vi "Test controller module.vi"(8 "error in (no error)":errorcluster) -> (0 "error out":errorcluster)   [LabVIEW 2016]
uses:
  Controls/Test controller modes.ctl
  Controls/Queue modes.ctl
  Controls/State control cluster.ctl
  Controls/States.ctl
  Actuator/Controls/Actuator fgv modes.ctl
  Actuator/Controls/Command cluster.ctl
  Actuator/Controls/Command list.ctl
  Controls/staus modes.ctl
  Webcam/Controls/Camera queue.ctl
  Webcam/Controls/Camera states.ctl
  DAQ/Controls/DAQ queue.ctl
  DAQ/Controls/Queue states.ctl
  Controls/data modes.ctl
  <vilib>/Utility/config.llb/NI_LVConfig.lvlib
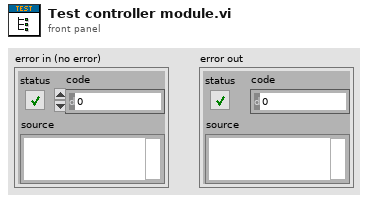
[diagram p1: front panel]
types:
  T1 = typedef "Queue modes.ctl" = enum16{"Initialise", "Destroy", "Get"}
  T2 = typedef "Test controller modes.ctl" = enum16{"Idle", "Test setup", "Check connections", "Populate FGV", "Load actuator settings", "Snap image", "Start move", "Start LC capture", "Wait", "Monitor", "Stop LC capture", "Save LC data", "Save Ivium data", "Save data"}
  T3 = typedef "References.ctl" = cluster{"Tab Control":refnum<vi>, "Logo 1":refnum<vi>, "Logo 2":refnum<vi>, "Connect Actuator":refnum<vi>, "LIVE DATA":refnum<vi>, "Speed":refnum<vi>, "Home position":refnum<vi>, "Limit position":refnum<vi>, "Trigger":refnum<vi>, "Current position":refnum<vi>, "Connect Camera":refnum<vi>, "TEST DATA":refnum<vi>, "LIVE DATA Force":refnum<vi>, "Connect DAQ":refnum<vi>, "Initialised":refnum<vi>, "Test":refnum<vi>}
  T4 = typedef "UEs.ctl" = cluster{"Read position":refnum<user-event>, "Check home":refnum<user-event>, "Record":refnum<user-event>, "Abort controller":refnum<user-event>, "Remote test":refnum<user-event>, "Test setup":refnum<user-event>, "Conditional wait":refnum<user-event>, "Abort move":refnum<user-event>, "Wait done":refnum<user-event>, "Send trigger":refnum<user-event>, "Initalising":refnum<user-event>, "Initalisation complete":refnum<user-event>}
  T5 = typedef "Command cluster.ctl" = cluster{"Command":T6, "data":variant}
  T6 = typedef "Command list.ctl" = enum16{"", "£nabort", "getaxisno", "£getserialno", "£nidentify", "&&£setnlimit", "&£nm", "&£snv", "&£speed", "£np", "£ncal"}
  T7 = typedef "Actuator fgv modes.ctl" = enum16{"Initalise", "COM", "Limit", "Speed", "Home", "Get"}
  T8 = typedef "State control cluster.ctl" = cluster{"State":T9, "Data":variant}
  T9 = typedef "States.ctl" = enum16{"Initialise", "Actuator connection", "Get info", "Send command", "Load method", "Run method", "Save test", "Setup", "Shutdown"}
  T10 = typedef "staus modes.ctl" = enum16{"Status", "Testing", "Webcam", "DAQ", "Actuator", "Initialise"}
  T11 = typedef "Camera queue.ctl" = cluster{"State":T12, "Data":variant}
  T12 = typedef "Camera states.ctl" = enum16{"Initialise", "Setup", "Connect", "Snap", "Close", "Shutdown"}
  T13 = typedef "DAQ queue.ctl" = cluster{"Sate":T14, "Data":variant}
  T14 = typedef "Queue states.ctl" = enum16{"Shutdown", "Save data", "Record", "Read", "Setup", "Zero", "Connect", "Initialise"}
  T15 = typedef "data modes.ctl" = enum16{"Initalise", "Status", "Process", "Add load", "Add position"}
  T16 = enum16{"open", "replace", "create", "open or create", "replace or create", "replace or create with confirmation"}
  T17 = typedef "Test settings.ctl" = cluster{"Speed (mm/s)":dbl, "Position limit":bool, "Position limit (mm)":dbl, "Load limit":bool, "Load limit (N)":dbl, "No. of repeats":u16, "Test identifier":string, "Time wait":bool, "Wait time (s)":dbl, "Trigger wait":bool, "Send trigger":bool, "Test notes":string, "Snap intervals":bool, "Time interval (s)":dbl}
  T18 = typedef "NI_LVConfig.lvlib/Config Data RefNum.ctl" = refnum<k1>
  T19 = typedef "Default settings.ctl" = cluster{"COM port":refnum<visa-resource-name>, "Home pos":dbl, "Speed":dbl, "Limit stop":dbl}
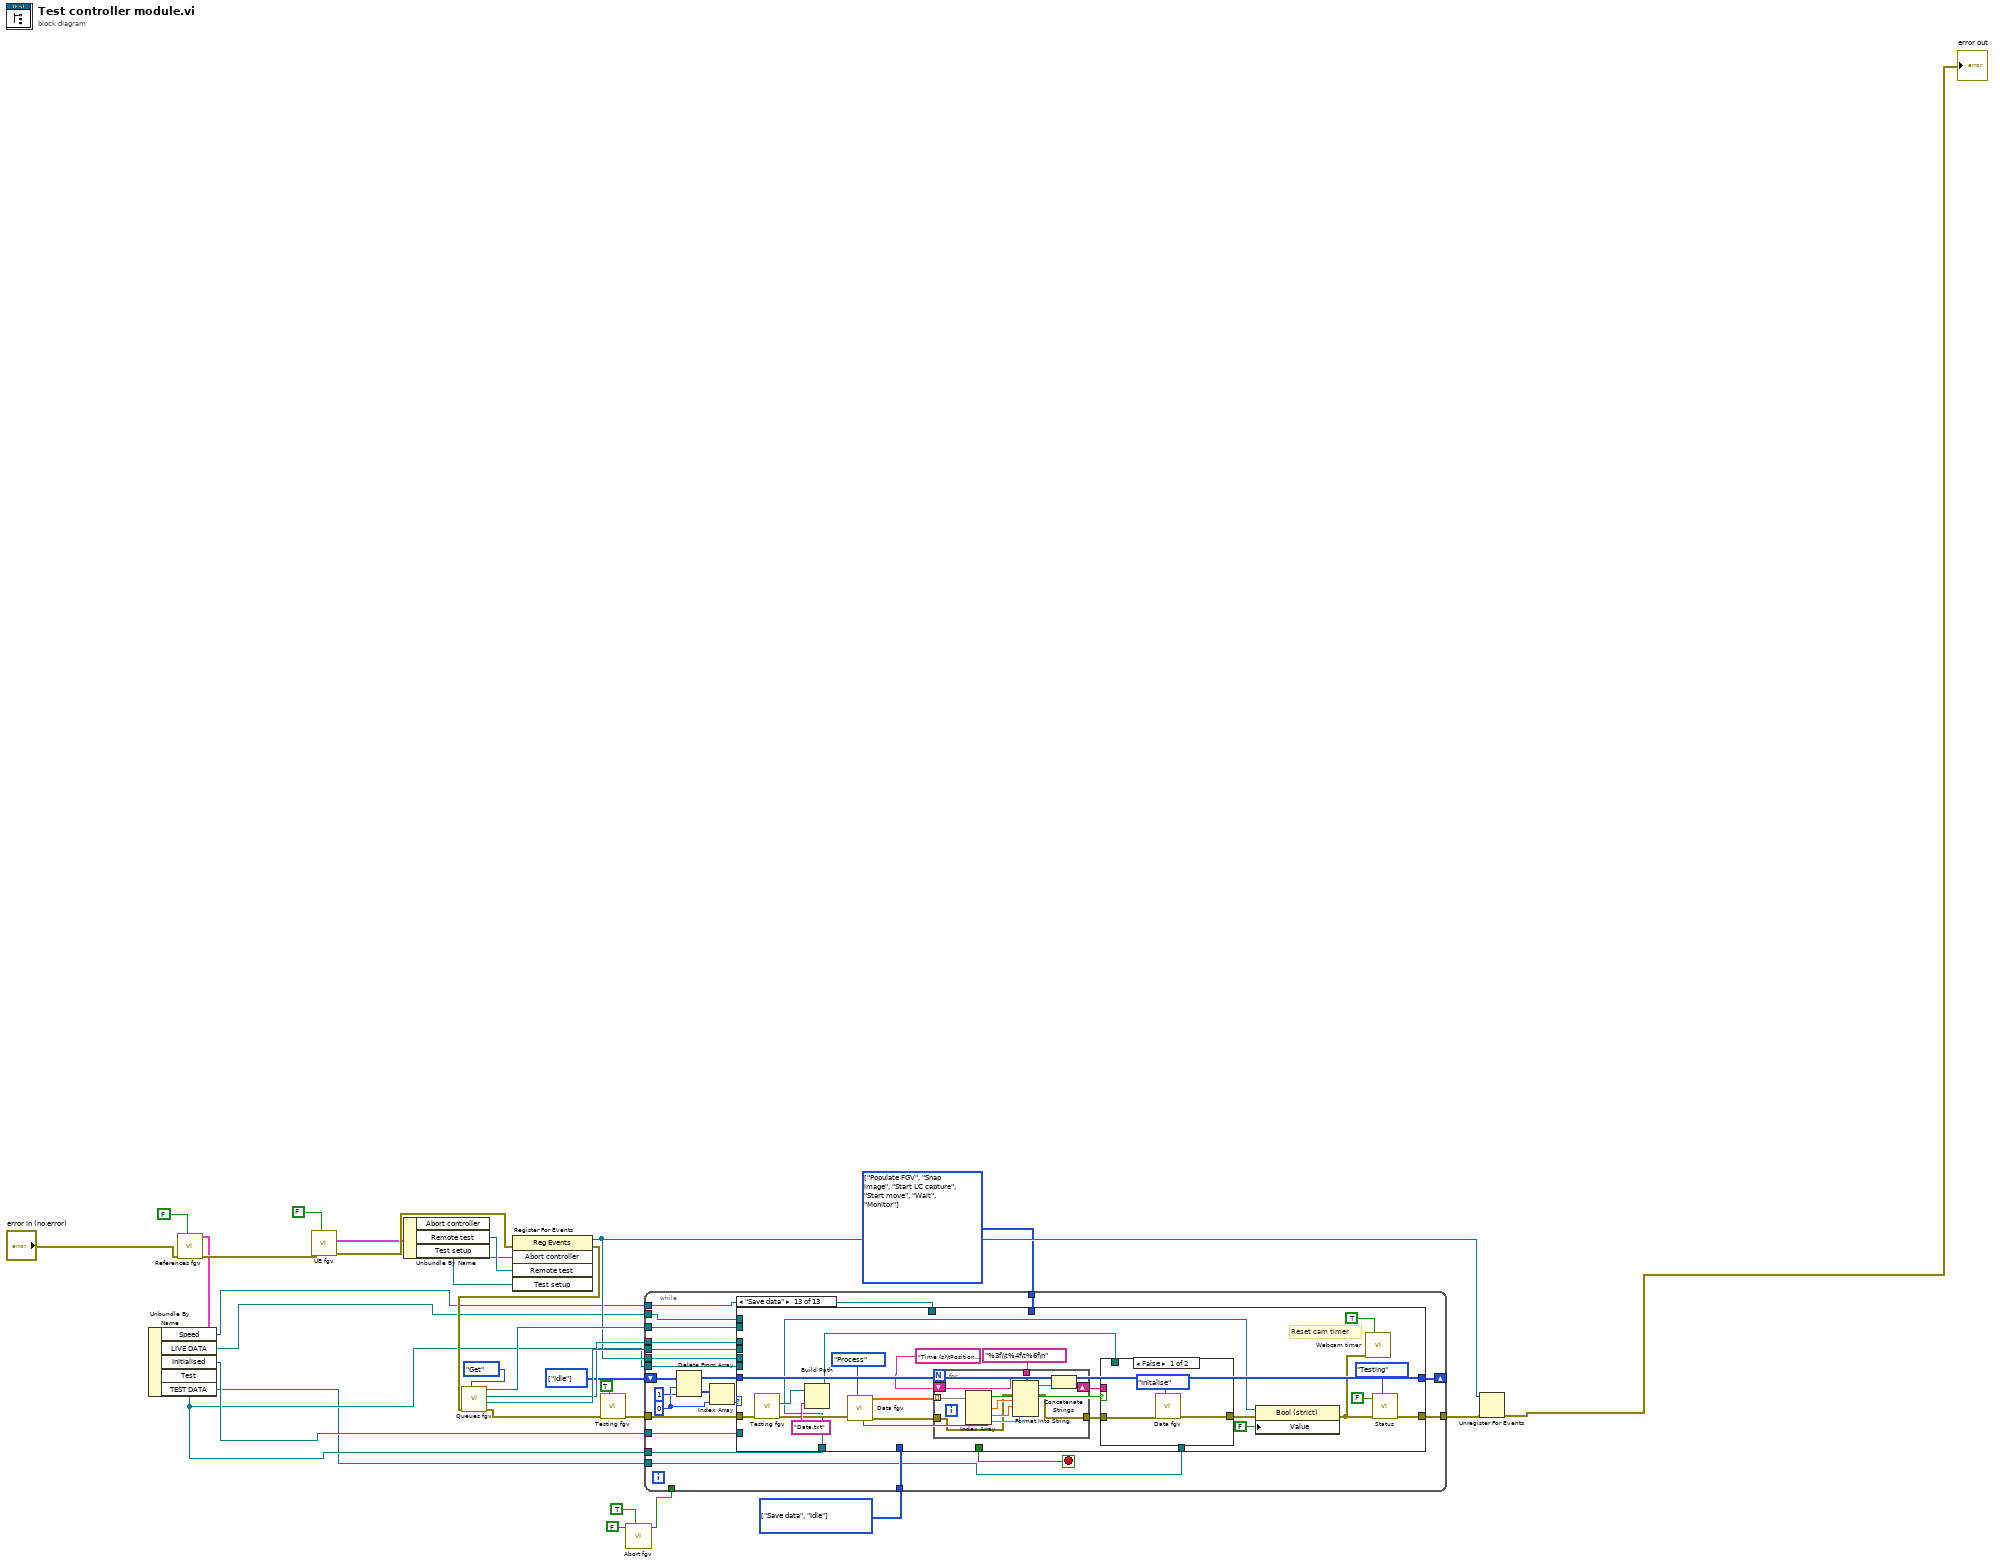
[diagram p0: block diagram]
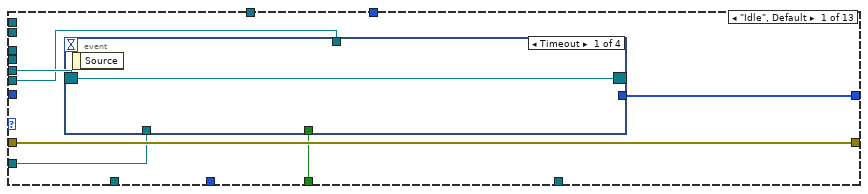
[diagram p2: hidden frame]
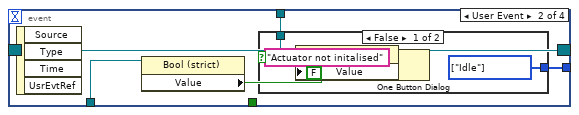
[diagram p3: hidden frame]
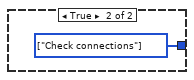
[diagram p4: hidden frame]
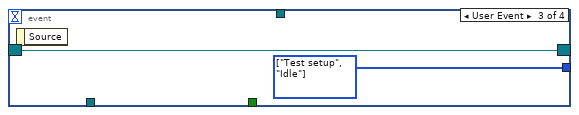
[diagram p5: hidden frame]
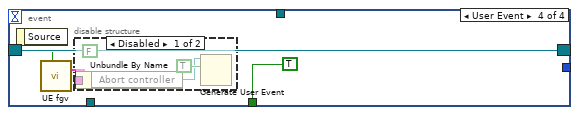
[diagram p6: hidden frame]
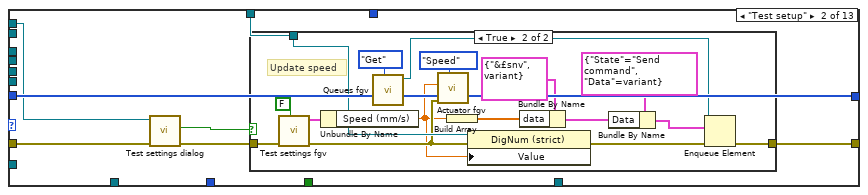
[diagram p8: hidden frame]
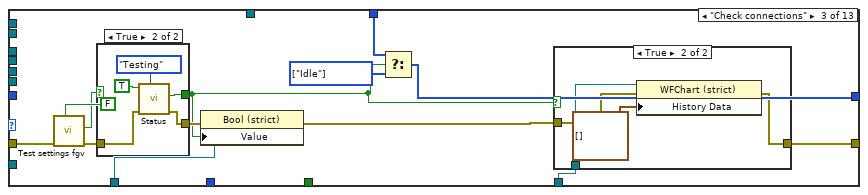
[diagram p10: hidden frame]
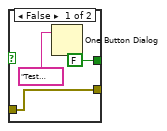
[diagram p12: hidden frame]
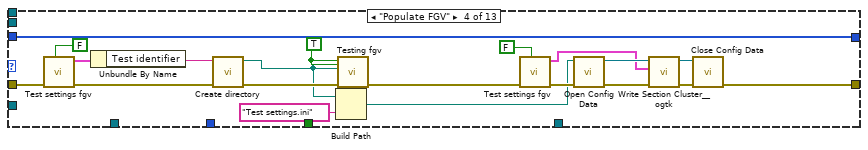
[diagram p13: hidden frame]
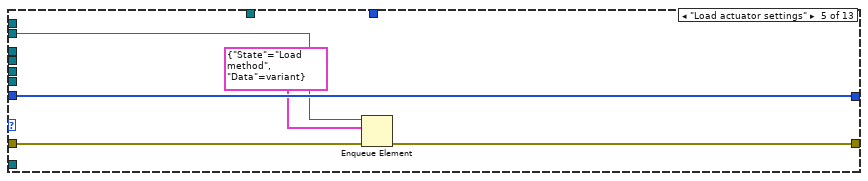
[diagram p14: hidden frame]
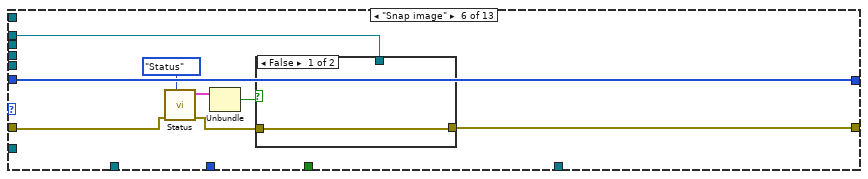
[diagram p15: hidden frame]
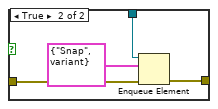
[diagram p16: hidden frame]
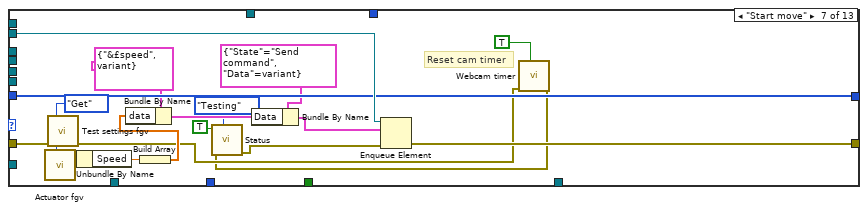
[diagram p17: hidden frame]
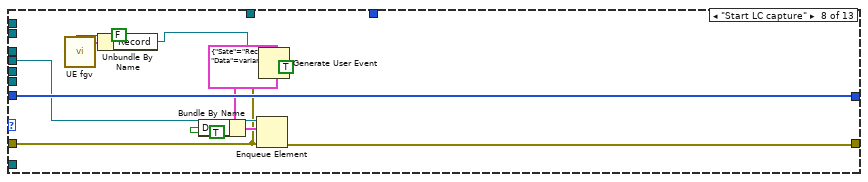
[diagram p18: hidden frame]
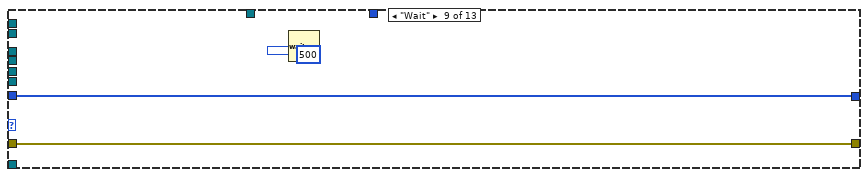
[diagram p19: hidden frame]
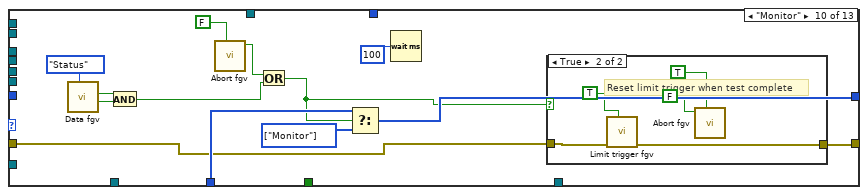
[diagram p20: hidden frame]
diagram:
  w15 = T2[] [enum."Save data", enum."Idle"] items=["Idle", "Test setup", "Check connections", "Populate FGV", "Load actuator settings", "Snap image", "Start move", "Start LC capture", "Wait", "Monitor", "Stop LC capture", "Save LC data", "Save Ivium data", "Save data"]
  w13 = T2[] [enum."Idle"] items=["Idle", "Test setup", "Check connections", "Populate FGV", "Load actuator settings", "Snap image", "Start move", "Start LC capture", "Wait", "Monitor", "Stop LC capture", "Save LC data", "Save Ivium data", "Save data"]
  w14 = T2[] [enum."Populate FGV", enum."Snap image", enum."Start LC capture", enum."Start move", enum."Wait", enum."Monitor"] items=["Idle", "Test setup", "Check connections", "Populate FGV", "Load actuator settings", "Snap image", "Start move", "Start LC capture", "Wait", "Monitor", "Stop LC capture", "Save LC data", "Save Ivium data", "Save data"]
  n1 = call "References fgv.vi"("Set?"=FALSE, "error in (no error)"="error in (no error)") -> ("error out"=w12:errorcluster, "Cluster"=w9:T3)  [unwired: 8 in]
  n2 = Unbundle By Name(w9) -> ("Speed"=w8:refnum<vi>, "LIVE DATA"=w7:refnum<vi>, "Initialised"=w6:refnum<vi>, "Test"=w5:refnum<vi>, "TEST DATA"=w4:refnum<vi>)
  n3 = call "UE fgv.vi"("Set?"=FALSE, "error in (no error)"=w12) -> ("error out"=w31:errorcluster, "UEs"=w27:T4)  [unwired: 7 in, 1 out]
  n4 = Unbundle By Name(w27) -> ("Abort controller"=w28:refnum<user-event>, "Remote test"=w29:refnum<user-event>, "Test setup"=w30:refnum<user-event>)
  n5 = register-events(error in=w31, w28, w29, w30) -> (reference out=w20:refnum<event-registration>, error out=w32:errorcluster)  [unwired: 1 in]
  n6 = call "Queues fgv.vi"("Modes"=Queue_modes."Get", "error in (no error)"=w32) -> ("error in (no error) 2"=w25:errorcluster, "DAQ"=w24:refnum<queue>, "Camera"=w23:refnum<queue>, "Ivium"=w22:refnum<queue>)  [unwired: 6 in]
  n7 = call "Testing fgv.vi"("Populate"=TRUE, "error in (no error)"=w25) -> ("error out"=w17:errorcluster)  [unwired: 7 in, 2 out]
  n8 = call "Abort fgv.vi"("Set?"=TRUE, "Value"=FALSE) -> ("Value 2"=w1:bool)  [unwired: 9 in]
  n9 = while {
    shift-right: [w49] -> _
    shift-left: w13 -> [w54]
    tunnel: w14 -> [w48]
    tunnel: w22 -> [w47]
    tunnel: w23 -> [w44]
    tunnel: [w46] -> w18
    tunnel: w17 -> [w45]
    tunnel: w15 -> [w43]
    tunnel: w24 -> [w41]
    tunnel: w20 -> [w40]
    tunnel: w5 -> [w38]
    tunnel: w7 -> [w37]
    tunnel: w8 -> [w36]
    tunnel: w6 -> [w35]
    tunnel: w5 -> [w34]
    tunnel: w4 -> [w33]
    tunnel: w1 -> [_]
    stop <- w39 stop-if-true
    w42 = 0 ("index")
    n10 = Delete From Array(array=w54, length=1, index=w42) -> (deleted portion=w52:T2[], array with subset deleted=w50:T2[])
    n11 = Index Array(array=w52, index=w42) -> (element=w51:T2)
    n12 = case shown="\"Save data\"" w51 {
      tunnel: w50 -> [_ w87 _ w150 w155 w162 w184 w197 w199 _ w230 w241 w263]
      tunnel: [w60 w87 w116 w150 w155 w162 w184 w197 w199 w210 w230 w241 w263] -> w49
      tunnel: w48 -> [_ _ w117 _ _ _ _ _ _ _ _ _ _]
      tunnel: w47 -> [_ _ _ _ w154 _ w185 _ _ _ _ _ _]
      tunnel: [w59 w82 w107 w131 w153 w163 w186 w192 w198 w205 w229 w239 w247] -> w46
      tunnel: w45 -> [w59 w86 w112 w147 w152 w158 w182 w191 w198 w206 w224 w236 w262]
      tunnel: w44 -> [_ _ _ _ _ w161 _ _ _ _ _ _ _]
      tunnel: w43 -> [_ _ _ _ _ _ _ _ _ w211 _ _ _]
      tunnel: w41 -> [_ _ _ _ _ _ _ w196 _ _ w228 w240 _]
      tunnel: w40 -> [w58 _ _ _ _ _ _ _ _ _ _ _ _]
      tunnel: [w57 _ _ _ _ _ _ _ _ _ _ _ _] -> w39
      tunnel: w38 -> [_ _ w114 _ _ _ _ _ _ _ _ _ w249]
      tunnel: w37 -> [_ w85 _ _ _ _ _ _ _ _ _ _ _]
      tunnel: w36 -> [_ w81 _ _ _ _ _ _ _ _ _ _ _]
      tunnel: w35 -> [w56 _ _ _ _ _ _ _ _ _ _ _ _]
      tunnel: w34 -> [w55 _ _ _ _ _ _ _ _ _ _ _ _]
      tunnel: w33 -> [_ _ w105 _ _ _ _ _ _ _ _ _ _]
      frame "Idle", Default {
        n13 = event shown="[0] Timeout" {
          selector: w58 -> [w61 w65 w73 w76]
          dyn-events: [w61 w65 w73 w76] -> _
          timeout: _ -> [_ _ _ _]
          tunnel: [_ w66 w72 _] -> w60
          tunnel: [_ _ _ TRUE] -> w57
          tunnel: w56 -> [_ w64 _ _]
          tunnel: w55 -> [_ w62 _ _]
          event Timeout {
            n14 = event-data() -> ()  [unwired: 1 in, 1 out]
          }
          event User Event {
            n15 = event-data() -> ()  [unwired: 1 in, 4 out]
            n16 = property class="Bool (strict)"(reference=w64) -> ("Value"=w63:bool)  [unwired: 1 in, 2 out]
            n17 = case shown="False" w63 {
              tunnel: [w70 w71] -> w66
              tunnel: w62 -> [w67 _]
              frame False {
                w70 = T2[] [enum."Idle"] items=["Idle", "Test setup", "Check connections", "Populate FGV", "Load actuator settings", "Snap image", "Start move", "Start LC capture", "Wait", "Monitor", "Stop LC capture", "Save LC data", "Save Ivium data", "Save data"]
                n18 = property on="Property Node" class="Bool (strict)"(reference=w67, "Value"=FALSE ("Test")) -> ()  [unwired: 1 in, 2 out]
                n19 = One Button Dialog(message="Actuator not initalised") -> ()  [unwired: 1 in, 1 out]
              }
              frame True {
                w71 = T2[] [enum."Check connections"] items=["Idle", "Test setup", "Check connections", "Populate FGV", "Load actuator settings", "Snap image", "Start move", "Start LC capture", "Wait", "Monitor", "Stop LC capture", "Save LC data", "Save Ivium data", "Save data"]
              }
            }
          }
          event User Event {
            w72 = T2[] [enum."Test setup", enum."Idle"] items=["Idle", "Test setup", "Check connections", "Populate FGV", "Load actuator settings", "Snap image", "Start move", "Start LC capture", "Wait", "Monitor", "Stop LC capture", "Save LC data", "Save Ivium data", "Save data"]
            n20 = event-data() -> ()  [unwired: 1 in, 1 out]
          }
          event User Event {
            n21 = event-data() -> ()  [unwired: 1 in, 1 out]
            n22 = call "UE fgv.vi"("Set?"=FALSE) -> ("UEs"=w74:T4)  [unwired: 8 in, 2 out]
            n23 = disable-structure shown="Disabled" {
              disable-tunnel: w74 -> [w79 _]
              frame Disabled {
                n24 = Unbundle By Name(w79) -> ("Abort controller"=w78:refnum<user-event>)
                n25 = Generate User Event(user event=w78, event data cluster=TRUE ("event data")) -> ()  [unwired: 2 in, 2 out]
              }
              frame Enabled {
              }
            }
          }
        }
      }
      frame "Test setup" {
        n26 = call "Test settings dialog.vi"("error in (no error)"=w86, "LIVE DATA 3"=w85) -> ("error out"=w83:errorcluster, "Confirmed"=w84:bool)  [unwired: 7 in, 1 out]
        n27 = case shown="True" w84 {
          tunnel: w83 -> [w88 w101]
          tunnel: [w88 w96] -> w82
          tunnel: w81 -> [_ w95]
          frame False {
          }
          frame True {
            # "Update speed"
            n28 = call "Test settings fgv.vi"("Set?"=FALSE, "error in (no error)"=w101) -> ("error out"=w94:errorcluster, "Test settings out"=w99:T17)  [unwired: 7 in, 1 out]
            n29 = Unbundle By Name(w99) -> ("Speed (mm/s)"=w90:dbl)
            n30 = call "Queues fgv.vi"("Modes"=Queue_modes."Get") -> ("Ivium"=w91:refnum<queue>)  [unwired: 7 in, 3 out]
            n31 = call "Actuator fgv.vi"("Enum"=Actuator_fgv_modes."Speed", "error in (no error)"=w94, "Data"=w90) -> ()  [unwired: 7 in, 2 out]
            n32 = Build Array(w90) -> (w89:dbl[])
            n33 = property class="DigNum (strict)"(reference=w95, error in=w94, "Value"=w90) -> (error out=w93:errorcluster)  [unwired: 1 out]
            n34 = Bundle By Name(cluster=T5 {"Command"=enum."&£snv", "data"=variant} ("Cluster"), "data"=w89) -> (w97:T5)
            n35 = Bundle By Name(cluster=T8 {"State"=enum."Send command", "Data"=variant} ("element"), "Data"=w97) -> (w103:T8)
            n36 = Enqueue Element(queue=w91, element=w103, error in (no error)=w93) -> (error out=w96:errorcluster)  [unwired: 1 in, 2 out]
          }
        }
      }
      frame "Check connections" {
        w115 = T2[] [enum."Idle"] items=["Idle", "Test setup", "Check connections", "Populate FGV", "Load actuator settings", "Snap image", "Start move", "Start LC capture", "Wait", "Monitor", "Stop LC capture", "Save LC data", "Save Ivium data", "Save data"] ("f")
        n37 = call "Test settings fgv.vi"("Set?"=FALSE, "error in (no error)"=w112) -> ("error out"=w111:errorcluster, "Settings selected?  out"=w109:bool)  [unwired: 7 in, 1 out]
        n38 = case shown="True" w109 {
          tunnel: [FALSE ("Testing") w130] -> w106
          tunnel: [w124 w129] -> w113
          tunnel: w111 -> [w124 w128]
          frame False {
            n39 = One Button Dialog(message="Test settings not selected.") -> ()  [unwired: 1 in, 1 out]
          }
          frame True {
            n40 = call "Status.vi"("Mode"=staus_modes."Testing", "error in (no error)"=w128, "Data"=TRUE) -> ("error out"=w129:errorcluster, "Testing"=w130:bool)  [unwired: 6 in, 1 out]
          }
        }
        n41 = property class="Bool (strict)"(reference=w114, error in=w113, "Value"=w106) -> (error out=w108:errorcluster)  [unwired: 1 out]
        n42 = Select(t=w117, s=w106, f=w115) -> (s? t:f=w116:T2[])
        n43 = case shown="True" w106 {
          tunnel: w108 -> [w118 w121]
          tunnel: [w118 w120] -> w107
          tunnel: w105 -> [_ w119]
          frame False {
          }
          frame True {
            n44 = property class="WFChart (strict)"(reference=w119, error in=w121, "History Data"=cluster{"Value":dbl, "data":dbl}[] []) -> (error out=w120:errorcluster)  [unwired: 1 out]
          }
        }
      }
      frame "Populate FGV" {
        w148 = TRUE ("Populate")
        n45 = call "Test settings fgv.vi"("Set?"=FALSE, "error in (no error)"=w147) -> ("error out"=w146:errorcluster, "Test settings out"=w144:T17)  [unwired: 7 in, 1 out]
        n46 = Unbundle By Name(w144) -> ("Test identifier"=w143:string)
        n47 = call "Create directory.vi"("error in (no error)"=w146, "Identifier 1"=w143) -> ("error out"=w149:errorcluster, "created path"=w135:path)  [unwired: 8 in]
        n48 = Build Path(base path=w135, name or relative path="Test settings.ini") -> (appended path=w133:path)
        n49 = call "Testing fgv.vi"("Populate"=w148, "error in (no error)"=w149, "test dir In"=w135, "Testing? In"=w148) -> ("error out"=w132:errorcluster)  [unwired: 5 in, 2 out]
        n50 = call "Test settings fgv.vi"("Set?"=FALSE, "error in (no error)"=w132) -> ("error out"=w138:errorcluster, "Test settings out"=w139:T17)  [unwired: 7 in, 1 out]
        n51 = call <vilib>:"Open Config Data.vi"("error in (no error)"=w138, "configuration file path"=w133) -> ("error out"=w137:errorcluster, "refnum"=w141:T18)  [unwired: 7 in, 1 out]
        n52 = call "Write Section Cluster__ogtk.vi"("error in (no error)"=w137, "Section Formatted Cluster"=w139, "refnum"=w141) -> ("error out"=w136:errorcluster, "dup refnum"=w142:T18)  [unwired: 7 in]
        n53 = call <vilib>:"Close Config Data.vi"("error in (no error)"=w136, "refnum"=w142) -> ("error out"=w131:errorcluster)  [unwired: 8 in, 1 out]
      }
      frame "Load actuator settings" {
        n54 = Enqueue Element(queue=w154, element=T8 {"State"=enum."Load method", "Data"=variant} ("State control"), error in (no error)=w152) -> (error out=w153:errorcluster)  [unwired: 1 in, 2 out]
      }
      frame "Snap image" {
        n55 = call "Status.vi"("Mode"=staus_modes."Status", "error in (no error)"=w158) -> ("error out"=w157:errorcluster, "Connections"=w160:cluster{"Data":bool, "Data":bool, "Data":bool})  [unwired: 7 in, 1 out]
        n56 = Unbundle(w160) -> ("Data"=w159:bool)  [unwired: 2 out]
        n57 = case shown="False" w159 {
          tunnel: [w164 w168] -> w163
          tunnel: w157 -> [w164 w167]
          tunnel: w161 -> [_ w165]
          frame False {
          }
          frame True {
            n58 = Enqueue Element(queue=w165, element=T11 {"State"=enum."Snap", "Data"=variant}, error in (no error)=w167) -> (error out=w168:errorcluster)  [unwired: 1 in, 2 out]
          }
        }
      }
      frame "Start move" {
        # "Reset cam timer"
        n59 = call "Actuator fgv.vi"("Enum"=Actuator_fgv_modes."Get") -> ("Cluster out"=w180:T19)  [unwired: 9 in, 1 out]
        n60 = call "Test settings fgv.vi"("error in (no error)"=w182) -> ("error out"=w171:errorcluster)  [unwired: 8 in, 2 out]
        n61 = Unbundle By Name(w180) -> ("Speed"=w179:dbl)
        n62 = Build Array(w179) -> (w178:dbl[])
        n63 = Bundle By Name(cluster=T5 {"Command"=enum."&£speed", "data"=variant} ("Cluster"), "data"=w178) -> (w177:T5)
        n64 = Bundle By Name(cluster=T8 {"State"=enum."Send command", "Data"=variant} ("State control"), "Data"=w177) -> (w175:T8)
        n65 = call "Webcam timer.vi"("Reset"=TRUE, "error in (no error)"=w171) -> ("error out"=w170:errorcluster)  [unwired: 7 in, 2 out]
        n66 = call "Status.vi"("Mode"=staus_modes."Testing", "error in (no error)"=w170, "Data"=TRUE) -> ("error out"=w172:errorcluster)  [unwired: 6 in, 2 out]
        n67 = Enqueue Element(queue=w185, element=w175, error in (no error)=w172) -> (error out=w186:errorcluster)  [unwired: 1 in, 2 out]
      }
      frame "Start LC capture" {
        n68 = call "UE fgv.vi"("Set?"=FALSE) -> ("UEs"=w189:T4)  [unwired: 8 in, 2 out]
        n69 = Unbundle By Name(w189) -> ("Record"=w187:refnum<user-event>)
        n70 = Bundle By Name(cluster=T13 {"Sate"=enum."Record", "Data"=variant} ("element"), "Data"=TRUE ("Test")) -> (w194:T13)
        n71 = Enqueue Element(queue=w196, element=w194, error in (no error)=w191) -> (error out=w192:errorcluster)  [unwired: 1 in, 2 out]
        n72 = Generate User Event(user event=w187, event data cluster=TRUE ("event data"), error in=w191) -> ()  [unwired: 1 in, 2 out]
      }
      frame "Wait" {
        n73 = Wait (ms)(milliseconds to wait=u32 500) -> ()  [unwired: 1 out]
      }
      frame "Monitor" {
        w212 = T2[] [enum."Monitor"] items=["Idle", "Test setup", "Check connections", "Populate FGV", "Load actuator settings", "Snap image", "Start move", "Start LC capture", "Wait", "Monitor", "Stop LC capture", "Save LC data", "Save Ivium data", "Save data"]
        n74 = call "Data fgv.vi"("Modes"=data_modes."Status") -> ("Load?"=w207:bool, "Position?"=w208:bool)  [unwired: 6 in, 3 out]
        n75 = And(x=w208, y=w207) -> (x .and. y?=w204:bool)
        n76 = call "Abort fgv.vi"("Set?"=FALSE) -> ("Value 2"=w202:bool)  [unwired: 10 in]
        n77 = Or(x=w202, y=w204) -> (x .or. y?=w203:bool)
        n78 = Select(t=w211, s=w203, f=w212) -> (s? t:f=w210:T2[])
        n79 = Wait (ms)(milliseconds to wait=u32 100) -> ()  [unwired: 1 out]
        n80 = case shown="True" w203 {
          tunnel: w206 -> [w214 w218]
          tunnel: [w214 w217] -> w205
          frame False {
          }
          frame True {
            # "Reset limit trigger when test complete"
            n81 = call "Limit trigger fgv.vi"("Reset"=TRUE, "error in (no error)"=w218) -> ("error out"=w217:errorcluster)  [unwired: 8 in, 1 out]
            n82 = call "Abort fgv.vi"("Set?"=TRUE, "Value"=FALSE ("Set?")) -> ()  [unwired: 9 in, 1 out]
          }
        }
      }
      frame "Stop LC capture" {
        n83 = Bundle By Name(cluster=T13 {"Sate"=enum."Record", "Data"=variant} ("element"), "Data"=FALSE) -> (w226:T13)
        n84 = call "UE fgv.vi"("Set?"=FALSE) -> ("UEs"=w222:T4)  [unwired: 8 in, 2 out]
        n85 = Enqueue Element(queue=w228, element=w226, error in (no error)=w224) -> (error out=w229:errorcluster)  [unwired: 1 in, 2 out]
        n86 = Unbundle By Name(w222) -> ("Record"=w220:refnum<user-event>)
        n87 = Generate User Event(user event=w220, event data cluster=FALSE ("event data"), error in=w224) -> ()  [unwired: 1 in, 2 out]
      }
      frame "Save LC data" {
        n88 = call "Testing fgv.vi"("Populate"=FALSE, "error in (no error)"=w236) -> ("error out"=w235:errorcluster, "test dir"=w234:path)  [unwired: 7 in, 1 out]
        n89 = Build Path(base path=w234, name or relative path="DAQ_data.txt") -> (appended path=w232:path)
        n90 = Bundle By Name(cluster=T13 {"Sate"=enum."Save data", "Data"=variant} ("element"), "Data"=w232) -> (w237:T13)
        n91 = Enqueue Element(queue=w240, element=w237, error in (no error)=w235) -> (error out=w239:errorcluster)  [unwired: 1 in, 2 out]
      }
      frame "Save data" {
        # "Reset cam timer"
        n92 = call "Testing fgv.vi"("error in (no error)"=w262) -> ("error out"=w253:errorcluster, "test dir"=w261:path)  [unwired: 8 in, 1 out]
        n93 = Build Path(base path=w261, name or relative path="Data.txt") -> (appended path=w255:path)
        n94 = call "Data fgv.vi"("Modes"=data_modes."Process", "error in (no error)"=w253) -> ("error out"=w252:errorcluster, "appended array"=w257:dbl[][], "Data"=w244:bool)  [unwired: 5 in, 2 out]
        n95 = for {
          tunnel: "%3f\\t%4f\t%6f\n" ("format string") -> [w285]
          shift-right: [w282] -> w254
          shift-left: "Time (s)\tPosition (mm)\tLoad (N)\n" ("format string") -> [w283]
          tunnel: w257 -> [w281] mode=indexing
          tunnel: w252 -> [w277]
          tunnel: [w276] -> w251
          n96 = Index Array(array=w281) -> (element #1=w280:dbl, element #2=w279:dbl, element #3=w278:dbl)  [unwired: 3 in]
          n97 = Format Into String(format string=w285, error in=w277, w280, w279, w278) -> (resulting string=w284:string, error out=w276:errorcluster)  [unwired: 1 in]
          n98 = Concatenate Strings(w283, w284) -> (w282:string)
        }
        n99 = case shown="False" w244 {
          tunnel: w255 -> [_ w272]
          tunnel: w254 -> [_ w270]
          tunnel: w251 -> [w266 w268]
          tunnel: [w264 w267] -> w250
          frame False {
            n100 = call "Data fgv.vi"("Modes"=data_modes."Initalise", "error in (no error)"=w266) -> ("error out"=w264:errorcluster)  [unwired: 5 in, 4 out]
          }
          frame True {
            n101 = Open/Create/Replace File(file path (use dialog)=w272, error in=w268, operation (0:open)=T16."create") -> (refnum out=w271:refnum<file>, error out=w269:errorcluster)  [unwired: 3 in, 1 out]
            n102 = Write to Text File(file (use dialog)=w271, text=w270, error in=w269) -> (refnum out=w275:refnum<file>, error out=w274:errorcluster)  [unwired: 1 in, 1 out]
            n103 = Close File(refnum=w275, error in=w274) -> (error out=w267:errorcluster)  [unwired: 1 out]
          }
        }
        n104 = property class="Bool (strict)"(reference=w249, error in=w250, "Value"=FALSE) -> (error out=w243:errorcluster)  [unwired: 1 out]
        n105 = call "Webcam timer.vi"("Reset"=TRUE, "error in (no error)"=w243) -> ()  [unwired: 7 in, 3 out]
        n106 = call "Status.vi"("Mode"=staus_modes."Testing", "error in (no error)"=w243, "Data"=FALSE) -> ("error out"=w247:errorcluster)  [unwired: 6 in, 2 out]
      }
    }
  }
  n107 = Unregister For Events(event registration refnum=w20, error in=w18) -> (error out=→"error out":errorcluster)
